vi "Read files T(Sequence).vi"(10 "Path":path, 11 "Number":dbl) -> (3 "Current":dbl format="%_1g")   [LabVIEW 2020, in "GPP.lvlib"]
uses:
  GPP.lvlib
panel:
  out "String":string
  out "String 2":string
  out "String 3":string
  out "Array":u8[](array[numeric])
  out "Numeric":u16
  out "T1":string
  out "Time":string
  out "LAST2":string
  out "Current":string
  out "LAST1":string
  out "Voltege":string
  out "ALL":string
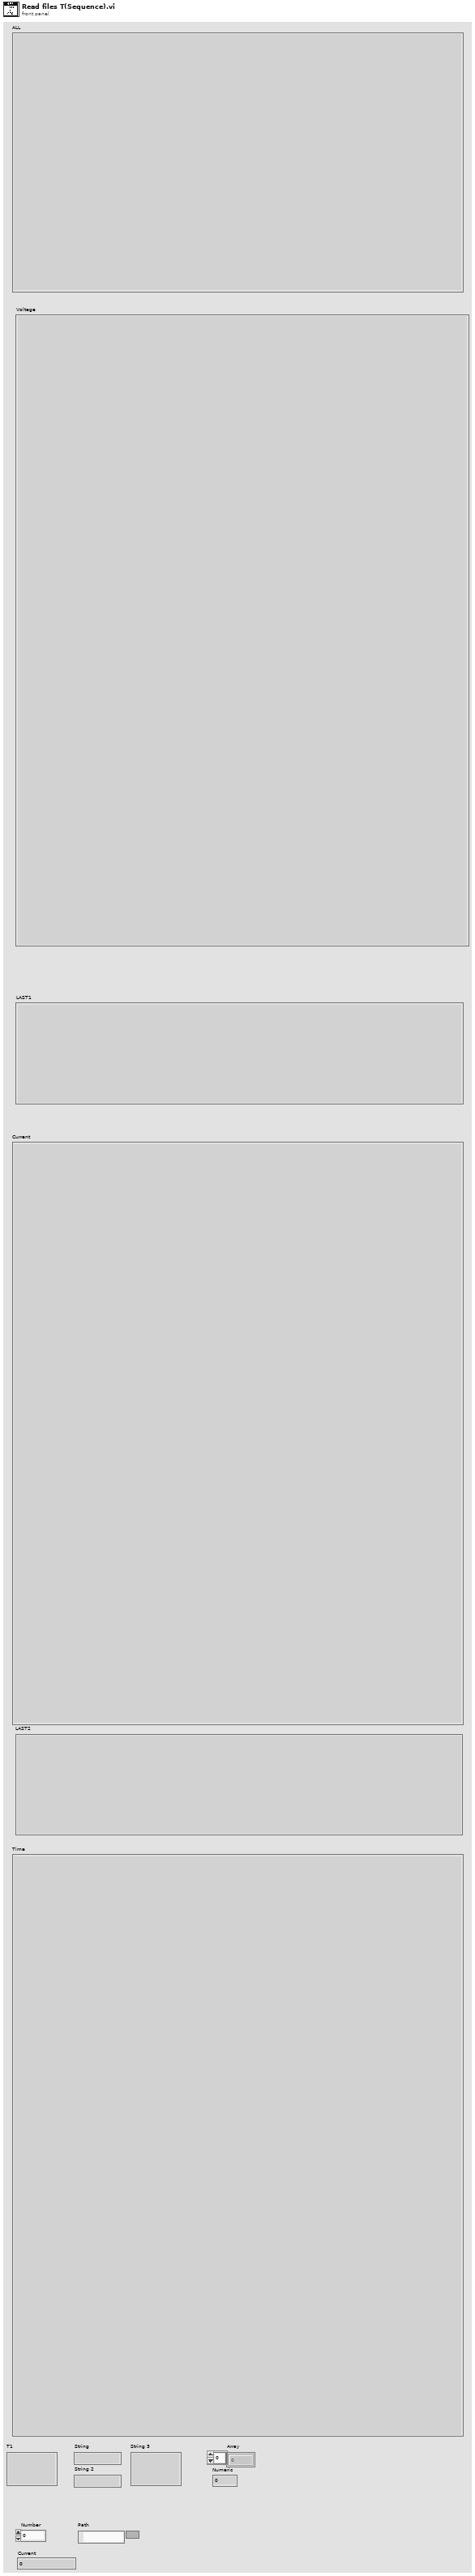
[diagram p1: front panel]
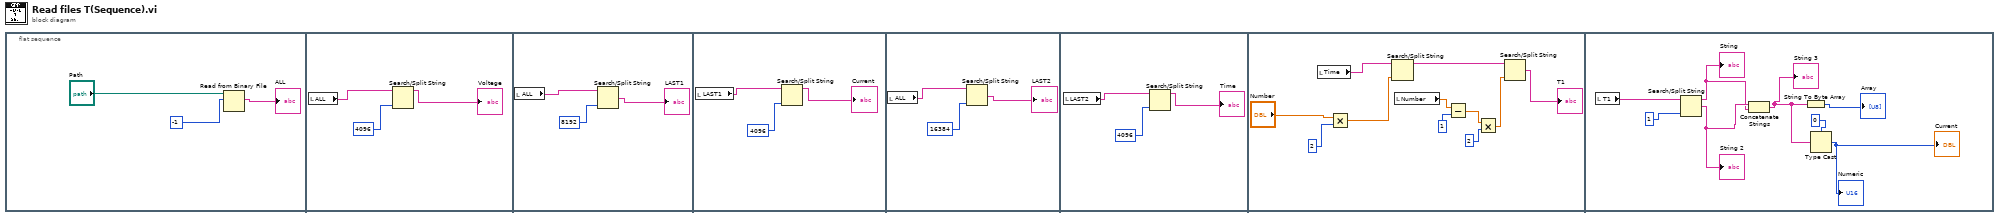
[diagram p0: block diagram]
diagram:
  n1 = flat-sequence {
    frame #0 {
      n2 = Read from Binary File(10:-1, 11:"Path") -> (2:→"ALL":string)  [unwired: 4 in, 3 out]
    }
    frame #1 {
      n3 = local read "ALL"() -> (w4:string)
      n4 = Search/Split String(string=w4, offset (0)=4096) -> (substring before match=→"Voltege":string)  [unwired: 1 in, 2 out]
    }
    frame #2 {
      n5 = local read "ALL"() -> (w7:string)
      n6 = Search/Split String(string=w7, offset (0)=8192) -> (match + rest of string=→"LAST1":string)  [unwired: 1 in, 2 out]
    }
    frame #3 {
      n7 = local read "LAST1"() -> (w10:string)
      n8 = Search/Split String(string=w10, offset (0)=4096) -> (substring before match=→"Current":string)  [unwired: 1 in, 2 out]
    }
    frame #4 {
      n9 = local read "ALL"() -> (w13:string)
      n10 = Search/Split String(string=w13, offset (0)=16384) -> (match + rest of string=→"LAST2":string)  [unwired: 1 in, 2 out]
    }
    frame #5 {
      n11 = local read "LAST2"() -> (w18:string)
      n12 = Search/Split String(string=w18, offset (0)=4096) -> (substring before match=→"Time":string)  [unwired: 1 in, 2 out]
    }
    frame #6 {
      n13 = local read "Time"() -> (w19:string)
      n14 = Multiply(x="Number", y=2) -> (x*y=w22:dbl)
      n15 = Search/Split String(string=w19, offset (0)=w22) -> (substring before match=w23:string)  [unwired: 1 in, 2 out]
      n16 = local read "Number"() -> (w25:dbl)
      n17 = Subtract(x=w25, y=1) -> (x-y=w26:dbl)
      n18 = Multiply(x=w26, y=2) -> (x*y=w28:dbl)
      n19 = Search/Split String(string=w23, offset (0)=w28) -> (match + rest of string=→"T1":string)  [unwired: 1 in, 2 out]
    }
    frame #7 {
      n20 = local read "T1"() -> (w31:string)
      n21 = Search/Split String(string=w31, offset (0)=1) -> (substring before match=w33:string, match + rest of string=w34:string)  [unwired: 1 in, 1 out]
      "String" <- w33
      "String 2" <- w34
      n22 = Concatenate Strings(w34, w33) -> (w36:string)
      "String 3" <- w36
      n23 = String To Byte Array(string=w36) -> (unsigned byte array=→"Array":u8[])
      n24 = Type Cast(type=u16 0, x=w36) -> (*(type *) &x=→"Numeric" →"Current":u16)
    }
  }
